vi "显示取像时间-右下角.vi"(9 "取像时间":u32, 11 "引用句柄输入":T1) -> (3 "Image Out":T1)   [LabVIEW 2014]
uses:
  <vilib>/vision/Image Controls.llb/IMAQ Image.ctl
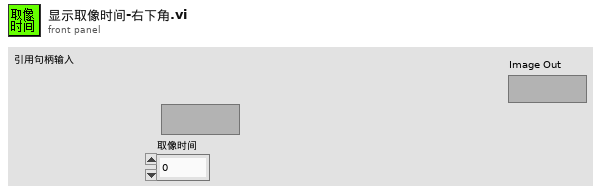
[diagram p1: front panel]
types:
  T1 = typedef "IMAQ Image.ctl" = refnum<image>
  T2 = cluster{"Desired Font (Application)":enum16{"User-specified Font", "Application Font", "System Font", "Dialog Font"}, "[User-specified Font]":cluster{"Font Name":string, "Size":i16, "Strikeout?":bool, "Italic?":bool, "Underline?":bool, "Outline?":bool, "Shadow?":bool, "Bold?":bool, "Rotation Angle":dbl}, "Horizontal Alignment":i16, "Vertical Alignment":i16}
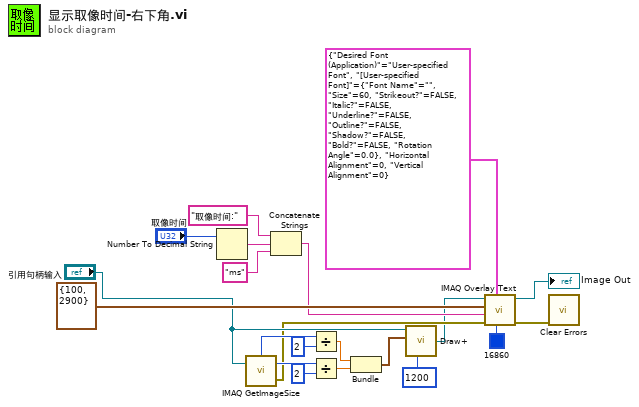
[diagram p0: block diagram]
diagram:
  n1 = Number To Decimal String(number="取像时间") -> (decimal integer string=w17:string)  [unwired: 1 in]
  n2 = call "IMAQ GetImageSize"("Image"="引用句柄输入") -> ("Y Resolution"=w6:i32, "X Resolution"=w9:i32, "error out"=w2:errorcluster)  [unwired: 3 in]
  n3 = Concatenate Strings("取像时间:" ("String"), w17, "ms" ("字符串")) -> (w16:string)
  n4 = Divide(x=w9, y=2) -> (x/y=w5:dbl)
  n5 = Divide(x=w6, y=2) -> (x/y=w4:dbl)
  n6 = Bundle(w5, w4) -> (w3:cluster{dbl, dbl})  [unwired: 1 in]
  n7 = call "Draw+.vi"("Width"=1200, "input cluster"=w3, "Image In"="引用句柄输入") -> ("Image Out"=w1:T1)  [unwired: 3 in]
  n8 = call "IMAQ Overlay Text"("Text Color (black)"=u32 16860, "Font, Size & Style"=T2 {"Desired Font (Application)"=enum."User-specified Font", "[User-specified Font]"={"Font Name"="", "Size"=60, "Strikeout?"=FALSE, "Italic?"=FALSE, "Underline?"=FALSE, "Outline?"=FALSE, "Shadow?"=FALSE, "Bold?"=FALSE, "Rotation Angle"=0.0}, "Horizontal Alignment"=0, "Vertical Alignment"=0}, "error in (no error)"=w2, "String"=w16, "Origin"=cluster{"X":i32, "Y":i32} {"X"=100, "Y"=2900}, "Image"=w1) -> ("error out"=w20:errorcluster, "Image Out"=→"Image Out":T1)  [unwired: 4 in]
  n9 = call <vilib>:"Clear Errors.vi"("error in (no error)"=w20) -> ()  [unwired: 5 in, 2 out]
